vi "cluster thamizh anish.vi"() -> ()   [LabVIEW 2011]
panel:
  in  "Numeric 7":dbl
  in  "Numeric 6":dbl
  in  "newe mark":dbl
  in  "sub no 1":dbl
  out "Cluster 7":T1
  in  "Cluster 6":T2
  out "Cluster 5":T3
  in  "Array 2":dbl[](array[numeric])
  out "Array":dbl[](array[numeric])
  in  "Cluster 4":T4
  out "Boolean 3":bool
  out "Numeric 5":dbl
  out "Numeric 2":dbl
  in  "Cluster 3":T5
  out "output 3":cluster{"Numeric":dbl, "Boolean":bool}
  in  "Boolean 2":bool
  in  "Numeric":dbl
  in  "Cluster 2":cluster{"Numeric":dbl, "Boolean":bool}
  out "Numeric 4":dbl
  out "Numeric 3":dbl
  out "Boolean":bool
  in  "Cluster":T6
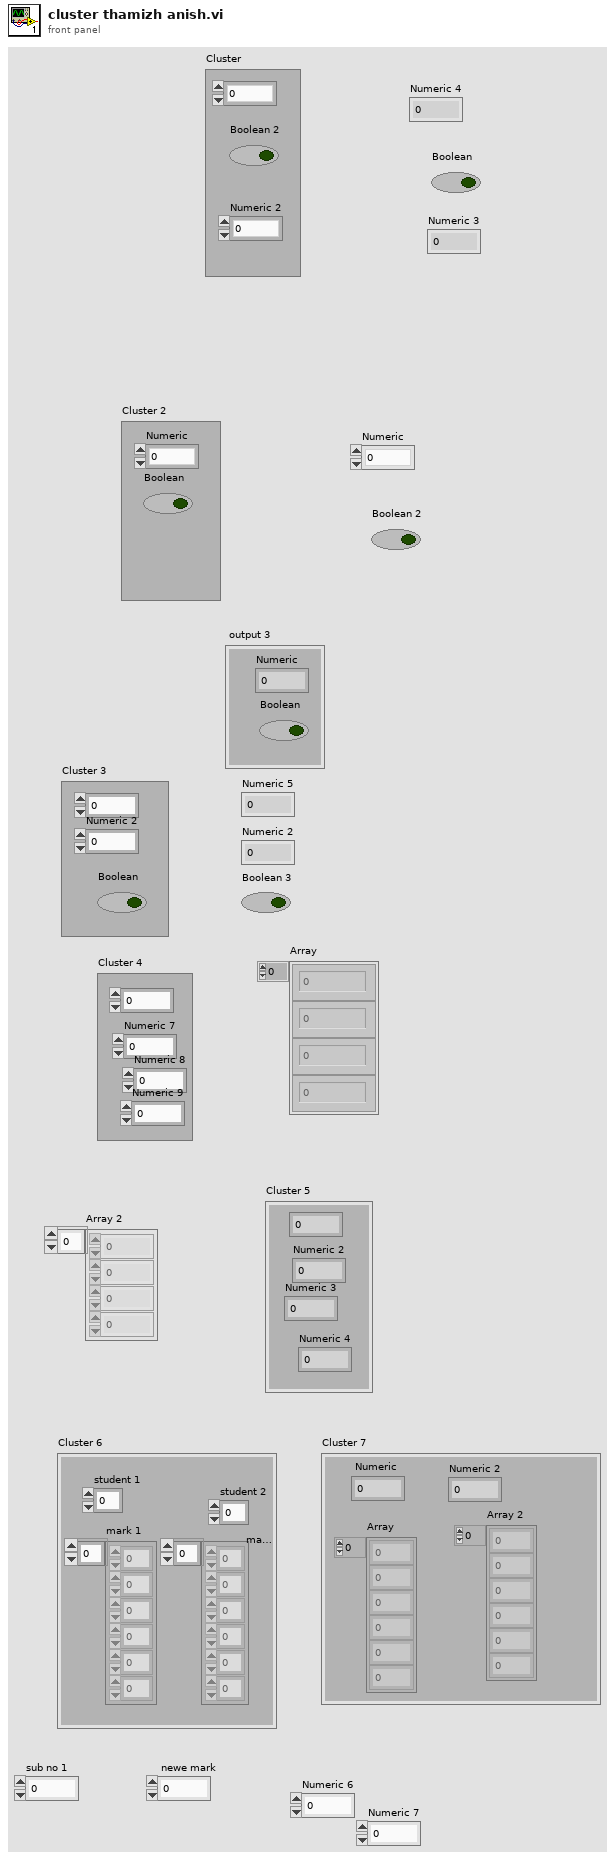
[diagram p1: front panel]
types:
  T1 = cluster{"Numeric":dbl, "Numeric 2":dbl, "Array":dbl[], "Array 2":dbl[]}
  T2 = cluster{"student 1":dbl, "student 2":dbl, "mark 1":dbl[], "mark 2":dbl[]}
  T3 = cluster{"Numeric":dbl, "Numeric 2":dbl, "Numeric 3":dbl, "Numeric 4":dbl}
  T4 = cluster{"Numeric 6":dbl, "Numeric 7":dbl, "Numeric 8":dbl, "Numeric 9":dbl}
  T5 = cluster{"Numeric":dbl, "Numeric 2":dbl, "Boolean":bool}
  T6 = cluster{"Boolean 2":bool, "Numeric 2":dbl, "Numeric":dbl}
  T7 = cluster{"Array 2[0]":dbl, "Array 2[1]":dbl, "Array 2[2]":dbl, "Array 2[3]":dbl}
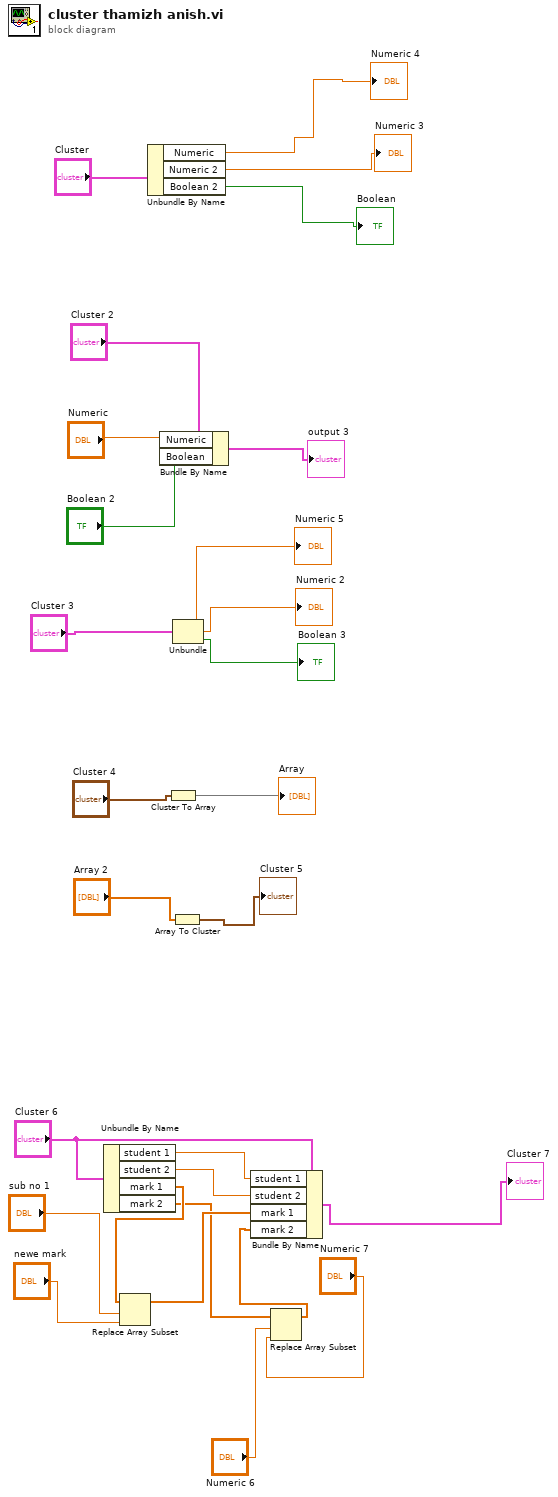
[diagram p0: block diagram]
diagram:
  n1 = Unbundle By Name("Cluster 6") -> ("student 1"=w5:dbl, "student 2"=w6:dbl, "mark 1"=w8:dbl[], "mark 2"=w4:dbl[])
  n2 = Replace Array Subset(array=w8, new element="newe mark", index="sub no 1") -> (w7:dbl[])
  n3 = Unbundle By Name("Cluster") -> ("Numeric"=→"Numeric 4":dbl, "Numeric 2"=→"Numeric 3":dbl, "Boolean 2"=→"Boolean":bool)
  n4 = Bundle By Name(cluster="Cluster 2", "Numeric"="Numeric", "Boolean"="Boolean 2") -> (→"output 3":cluster{"Numeric":dbl, "Boolean":bool})
  n5 = Cluster To Array(cluster="Cluster 4") -> (array=→"Array":dbl[])
  n6 = Array To Cluster(array="Array 2") -> (cluster=→"Cluster 5":T7)
  n7 = Unbundle("Cluster 3") -> ("Numeric"=→"Numeric 5":dbl, "Numeric 2"=→"Numeric 2":dbl, "Boolean"=→"Boolean 3":bool)
  n8 = Replace Array Subset(array=w4, new element="Numeric 7", index="Numeric 6") -> (w1:dbl[])
  n9 = Bundle By Name(cluster="Cluster 6", "student 1"=w5, "student 2"=w6, "mark 1"=w7, "mark 2"=w1) -> (→"Cluster 7":T2)
